vi "logon tcp.vi"(8 "error in":errorcluster, 10 "Data Servers":string[](array[string])=["dataserver.cee.cornell.edu", "calcium.cee.cornell.edu"], 11 "port":u16=6341) -> (0 "error out":errorcluster, 1 "Server stats":T1={"scan rate"=10.0, "# connections"=0, "channel settings"=[]} {"channel settings"."lower input limits" format="%.4f"; "channel settings"."upper input limits" format="%.4f"; "scan rate" format="%.2f"}, 2 "data server address":string="128.84.245.227", 3 "connection ID":refnum<k5>, 4 "restart":bool, 5 "Data Servers out":string[](array[string])=["calcium.cee.cornell.edu", "Dataserver.cee.cornell.edu"])   [LabVIEW 2012]
doc: "Open data server opens a connection with a data server. If the array of data servers contains only one element then the connection is made immediately. If the array contains more than one element a subvi with a dialog box opens to select the data server. TCP is then used to log on to the data server and data server information is returned in the Server Stats control.\n\nInputs\n\nPort - TCP port number. Must be the same as the port number used by the data server. At Cornell CEE we use port 6341.\n\nData Servers - An array of strings that are either names or IP addresses for available dataservers \n\nError in - \n\nOutputs\n\nData server address - String containing the name or the IP address of the selected data server.\n\nRestart - Boolean that is true if the connection with the data server could not be established.\n\nServer Stats - Data server information including scan rate, number of client connections and channel information.\n\nError out - \n\n\nCreated by Monroe Weber-Shirk\nCornell University\nmw24@cornell.edu\nJanuary 2000"
uses:
  DataServer/Server stats.ctl
panel:
  # "Hz"
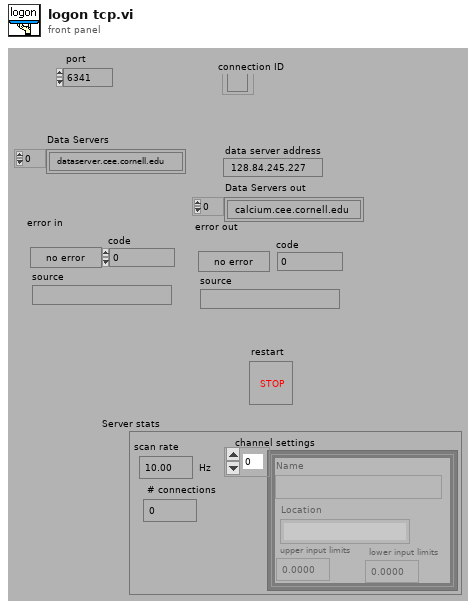
[diagram p1: front panel]
types:
  T1 = typedef "Server stats.ctl" = cluster{"scan rate":dbl, "# connections":i32, "channel settings":cluster{"Name":string, "upper input limits":sgl, "lower input limits":sgl, "Location":string}[]}
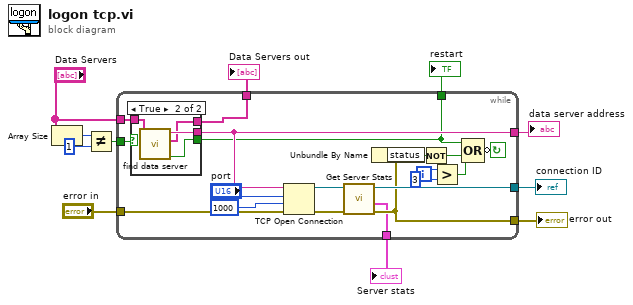
[diagram p0: block diagram]
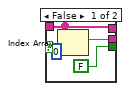
[diagram p2: hidden frame]
diagram:
  n1 = Array Size(array="Data Servers") -> (size(s)=w5:i32)
  n2 = Not Equal?(x=w5, y=1) -> (x != y?=w3:bool)
  n3 = while {
    tunnel: [w13] -> w2
    tunnel: w3 -> [w14]
    tunnel: "error in" -> [w21]
    tunnel: [w22] -> w8
    tunnel: [w27] -> w9
    tunnel: [w23] -> w10
    tunnel: [w19] -> w11
    tunnel: "Data Servers" -> [w25]
    tunnel: [w12] -> w1
    i -> [w17]
    stop <- w20 continue-if-true
    n4 = case shown="True" w14 {
      tunnel: w25 -> [w31 w38]
      tunnel: [w33 w37] -> w23
      tunnel: [FALSE w36] -> w19
      tunnel: [w31 w35] -> w13
      frame False {
        n5 = Index Array(array=w31, index=0 ("Index")) -> (element=w33:string)
      }
      frame True {
        n6 = call "find data server.vi"("Data Servers"=w38) -> ("Restart"=w36:bool, "Data Servers out"=w35:string[], "data server address out"=w37:string)  [unwired: 8 in]
      }
    }
    n7 = TCP Open Connection(address=w23, remote port or service name="port", timeout ms (60000)=1000, error in (no error)=w21) -> (connection ID=w28:refnum<k5>, error out=w29:errorcluster)  [unwired: 1 in]
    n8 = call "Get Server Stats.vi"("error in (no error)"=w29, "Connection ID"=w28) -> ("error out"=w22:errorcluster, "Server stats"=w12:T1, "Connection ID"=w27:refnum<k5>)  [unwired: 6 in, 1 out]
    n9 = Unbundle By Name(w22) -> ("status"=w24:bool)
    n10 = Not(x=w24) -> (.not. x?=w18:bool)
    n11 = Greater?(x=w17, y=3) -> (0:w15:bool)
    n12 = Compound Arithmetic op=OR(w19, w18, w15) -> (invert w20:bool)
  }
  "data server address" <- w10
  "restart" <- w11
  "connection ID" <- w9
  "error out" <- w8
  "Data Servers out" <- w2
  "Server stats" <- w1
